vi "magnet global state.vi"(8 "input cluster":T1, 10 "initialized":bool, 11 "magnet global state action":T2) -> (0 "output cluster":T1, 3 "initialized":bool)   [LabVIEW 2013]
uses:
  magnet global state action.ctl
  magnet global state.ctl
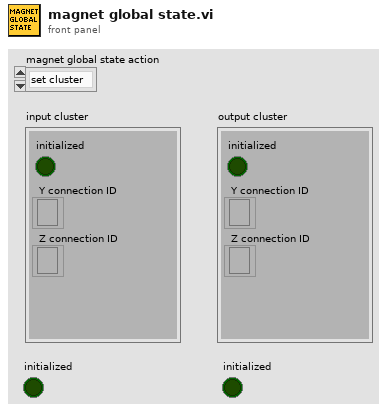
[diagram p1: front panel]
types:
  T1 = typedef "magnet global state.ctl" = cluster{"initialized":bool, "Y connection ID":refnum<k5>, "Z connection ID":refnum<k5>}
  T2 = typedef "magnet global state action.ctl" = enum16{"set cluster", "get cluster", "set initialized", "get initialized"}
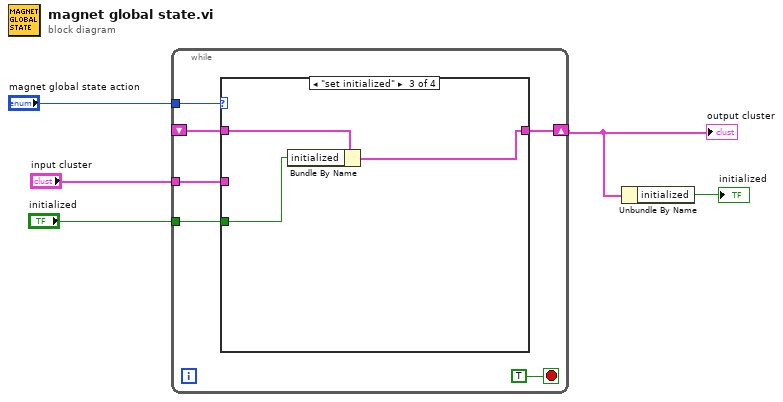
[diagram p0: block diagram]
diagram:
  n1 = while {
    tunnel: "magnet global state action" -> [w10]
    shift-right: [w8] -> w2
    shift-left: _ -> [w7]
    tunnel: "input cluster" -> [w9]
    tunnel: "initialized" -> [w6]
    stop <- TRUE stop-if-true
    n2 = case shown="\"set initialized\"" w10 {
      tunnel: w9 -> [w12 _ _ _]
      tunnel: [w12 w13 w14 w17] -> w8
      tunnel: w7 -> [_ w13 w16 w17]
      tunnel: w6 -> [_ _ w15 _]
      frame "set cluster", Default {
      }
      frame "get cluster" {
      }
      frame "set initialized" {
        n3 = Bundle By Name(cluster=w16, "initialized"=w15) -> (w14:T1)
      }
      frame "get initialized" {
      }
    }
  }
  "output cluster" <- w2
  n4 = Unbundle By Name(w2) -> ("initialized"=→"initialized":bool)
